vi "Convex Hull 3D (GiftWrap) example.vi"(0 "Points":sgl[][](array[numeric])=[[0.0, 0.0, 0.0], [1.0, 0.0, 0.0], [1.0, 1.0, 0.0], [0.0, 1.0, 0.0], [0.0, 0.0, 1.0], [1.0, 0.0, 1.0], [1.0, 1.0, 1.0], [0.0, 1.0, 1.0], [10.0, 10.0, 0.0], [11.0, 10.0, 0.0], [11.0, 11.0, 0.0], [10.0, 11.0, 0.0], [10.0, 10.0, 1.0], [11.0, 10.0, 1.0], [11.0, 11.0, 1.0], [10.0, 11.0, 1.0]]) -> (1 "Convex hull triangles (partial proc.)":T1[](array[typedef]), 2 "Stack error":errorcluster)   [LabVIEW 2014]
uses:
  Typedefs/Triangle.ctl
  <vilib>/Utility/miscctls.llb/LVRGBAColorTypeDef.ctl
panel:
  in  "Delaunay":bool=TRUE
  in  "Render mode":T2(ring)=enum."Wireframe"
  out "3D Picture":refnum<vi>(3d-picture)
  in  "Random start pts":bool=TRUE
  in  "Npts random":i32=32
  # "PN 21/03/2015"
  # "Vertices"
  # "Edges"
  # "Unit normal"
  # "Edge unit normals"
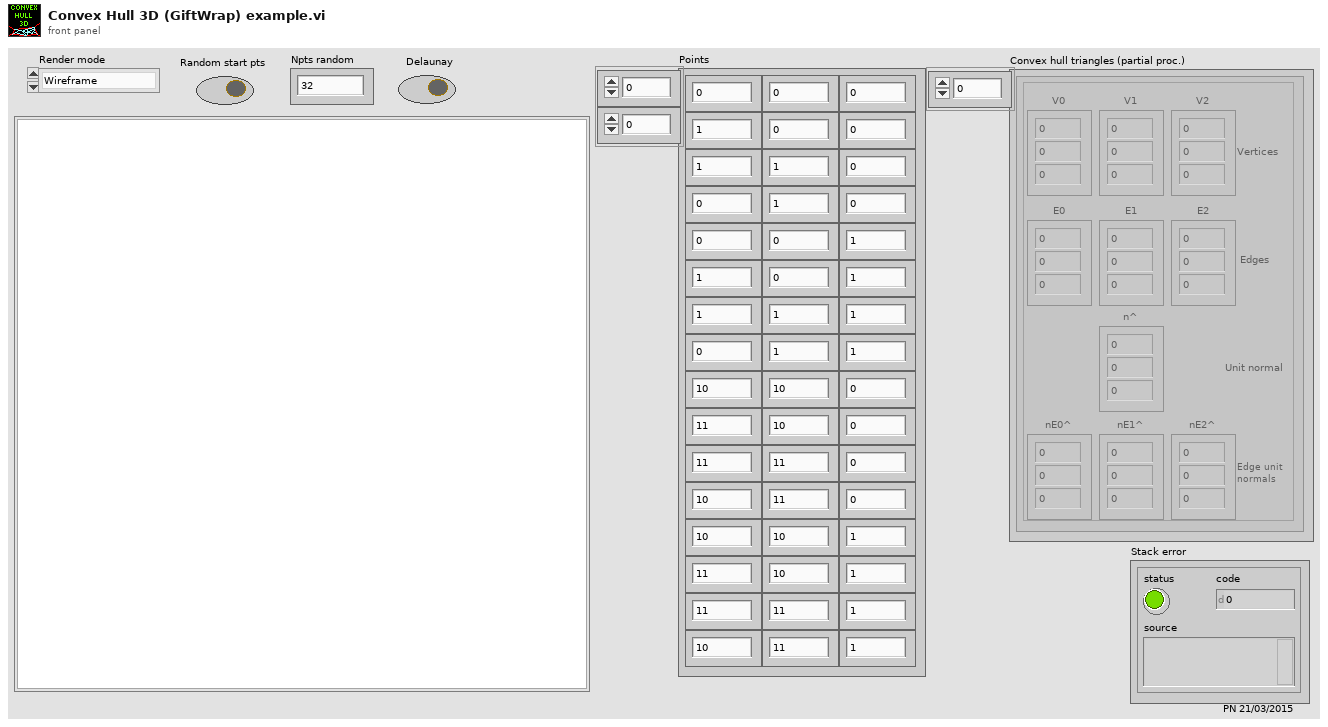
[diagram p1: front panel]
types:
  T1 = typedef "Triangle.ctl" = cluster{"V0":sgl[], "V1":sgl[], "V2":sgl[], "E0":sgl[], "E1":sgl[], "E2":sgl[], "n^":sgl[], "nE0^":sgl[], "nE1^":sgl[], "nE2^":sgl[]}
  T2 = enum16{"Inherit Value", "Points", "Wireframe", "Polygons"}
  T3 = cluster{"Red":sgl, "Green":sgl, "Blue":sgl, "Alpha":sgl}
  T4 = typedef "LVRGBAColorTypeDef.ctl" = cluster{"Red":sgl, "Green":sgl, "Blue":sgl, "Alpha":sgl}
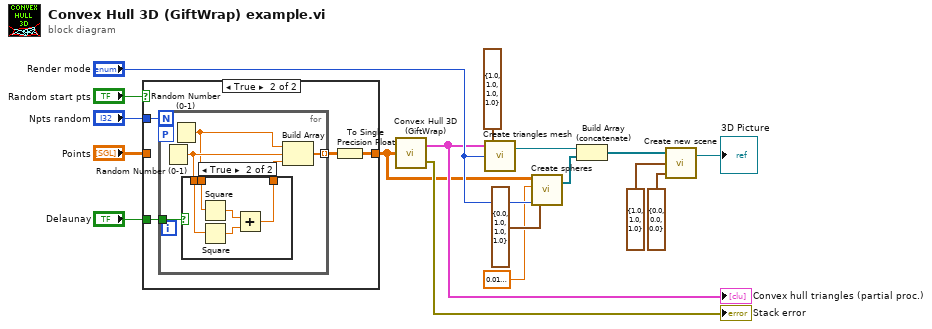
[diagram p0: block diagram]
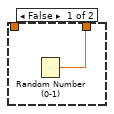
[diagram p3: hidden frame]
diagram:
  n1 = case shown="True" "Random start pts" {
    tunnel: "Npts random" -> [_ w22]
    tunnel: "Points" -> [w18 _]
    tunnel: [w18 w20] -> w1
    tunnel: "Delaunay" -> [_ w19]
    frame False {
    }
    frame True {
      n2 = for {
        N: w22 -> [_]
        tunnel: [w27] -> w21 mode=indexing
        workers-P: _ -> [_]
        tunnel: w19 -> [w26]
        n3 = Random Number (0-1)() -> (number: 0 to 1=w24:dbl)
        n4 = Random Number (0-1)() -> (number: 0 to 1=w23:dbl)
        n5 = case shown="True" w26 {
          tunnel: [w28 w31] -> w25
          tunnel: w24 -> [_ w30]
          tunnel: w23 -> [_ w29]
          frame False {
            n6 = Random Number (0-1)() -> (number: 0 to 1=w28:dbl)
          }
          frame True {
            n7 = Square(x=w29) -> (x^2=w33:dbl)
            n8 = Square(x=w30) -> (x^2=w32:dbl)
            n9 = Add(x=w33, y=w32) -> (x+y=w31:dbl)
          }
        }
        n10 = Build Array(w23, w24, w25) -> (w27:dbl[])
      }
      n11 = To Single Precision Float(number=w21) -> (single precision float=w20:sgl[][])
    }
  }
  n12 = call "Convex Hull 3D (GiftWrap).vi"("Vertices"=w1) -> ("Convex hull triangles (partial proc.)"=w4:T1[], "Stack error"=→"Stack error":errorcluster)
  "Convex hull triangles (partial proc.)" <- w4
  n13 = call "Create triangles mesh.vi"("Colour"=T4 {"Red"=1.0, "Green"=1.0, "Blue"=1.0, "Alpha"=1.0}, "Render mode"="Render mode", "Triangles array"=w4) -> ("Triangle mesh out"=w14:refnum<vi>)  [unwired: 1 out]
  n14 = call "Create spheres.vi"("Render mode"="Render mode", "Colour"=T3 {"Red"=0.0, "Green"=1.0, "Blue"=1.0, "Alpha"=1.0}, "Radius (model units)"=sgl 0.02, "Points array"=w1) -> ("Points"=w6:refnum<vi>[])  [unwired: 1 out]
  n15 = Build Array (concatenate)(w14, w6) -> (w13:refnum<vi>[])
  n16 = call "Create new scene.vi"("Translation"=cluster{"X":sgl, "Y":sgl, "Z":sgl} {"X"=0.0, "Y"=0.0, "Z"=0.0}, "Scale"=cluster{"X":sgl, "Y":sgl, "Z":sgl} {"X"=1.0, "Y"=1.0, "Z"=1.0}, "Scene objects array"=w13) -> ("Scene out"=→"3D Picture":refnum<vi>)  [unwired: 1 out]
